vi "client.vi"() -> ()   [LabVIEW 2013]
panel:
  out "Waveform Graph":dbl[](graph)
  out "data out":string
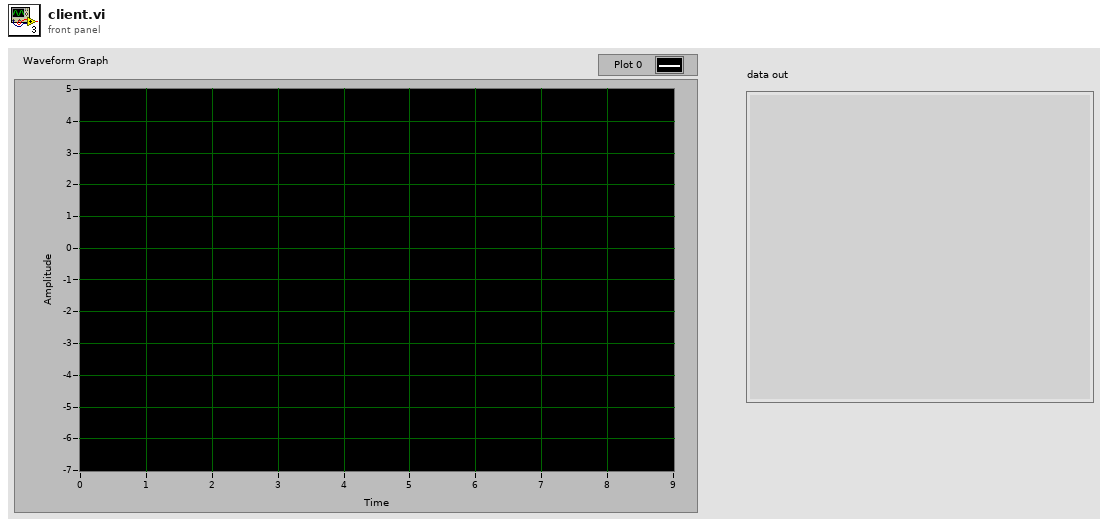
[diagram p1: front panel]
types:
  T1 = enum16{"Standard", "Buffered", "CRLF", "Immediate"}
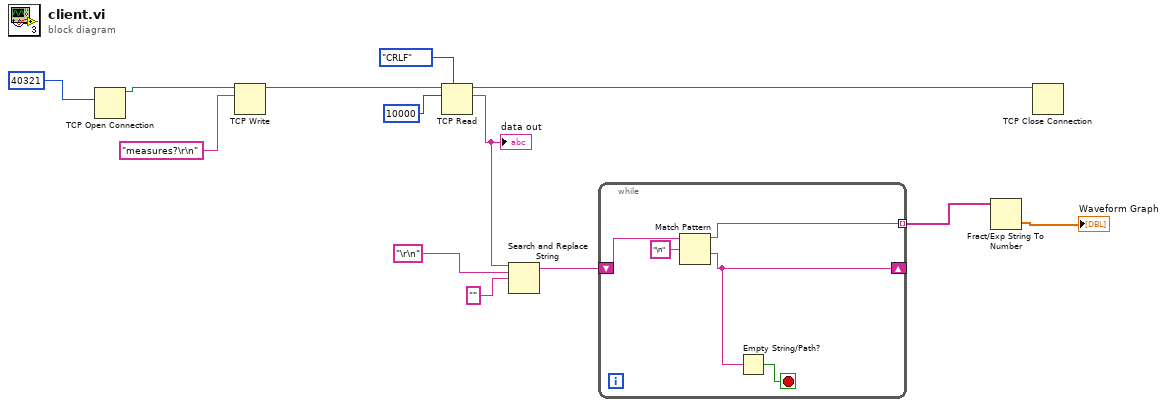
[diagram p0: block diagram]
diagram:
  n1 = TCP Open Connection(remote port or service name=u16 40321) -> (connection ID=w12:refnum<k5>)  [unwired: 4 in, 1 out]
  n2 = TCP Write(connection ID=w12, data in="measures?\r\n") -> (connection ID out=w10:refnum<k5>)  [unwired: 2 in, 2 out]
  n3 = TCP Read(connection ID=w10, bytes to read=10000, 7:T1."CRLF" ("mode (standard)")) -> (connection ID out=w7:refnum<k5>, data out=w5:string)  [unwired: 2 in, 1 out]
  "data out" <- w5
  n4 = Search and Replace String(input string=w5, search string="\r\n", replace string="" ("replace string (\"\")")) -> (result string=w6:string)  [unwired: 5 in, 3 out]
  n5 = while {
    shift-right: [w16] -> _
    shift-left: w6 -> [w18]
    tunnel: [w14] -> w2 mode=indexing
    stop <- w15 stop-if-true
    n6 = Match Pattern(string=w18, regular expression="\n") -> (before substring=w14:string, after substring=w16:string)  [unwired: 1 in, 2 out]
    n7 = Empty String/Path?(string/path=w16) -> (empty?=w15:bool)
  }
  n8 = Fract/Exp String To Number(string=w2) -> (number=→"Waveform Graph":dbl[])  [unwired: 3 in, 1 out]
  n9 = TCP Close Connection(connection ID=w7) -> ()  [unwired: 2 in, 2 out]
